vi "create_pattern.vi"(7 "sampling rate":dbl[unit], 8 "error in (no error)":errorcluster, 9 "duration":dbl[unit], 10 "amplitude":dbl, 11 "frequency":dbl[unit]=20000.0) -> (0 "error out":errorcluster, 2 "pattern values":dbl[](array[numeric]))   [LabVIEW 2010]
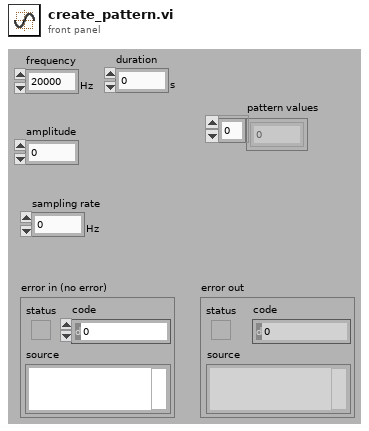
[diagram p1: front panel]
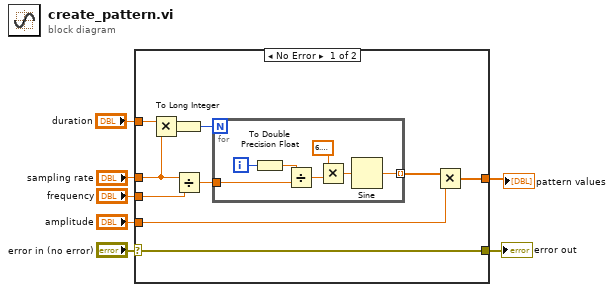
[diagram p0: block diagram]
diagram:
  n1 = case shown="No Error" "error in (no error)" {
    selector: "error in (no error)" -> [w17 w25]
    tunnel: [w17 w25] -> w6
    tunnel: "amplitude" -> [w16 _]
    tunnel: "frequency" -> [w13 _]
    tunnel: [w14 _] -> w3
    tunnel: "sampling rate" -> [w10 _]
    tunnel: "duration" -> [w11 _]
    frame No Error {
      n2 = Multiply(x=w11, y=w10) -> (x*y=w9:dbl)
      n3 = To Long Integer(number=w9) -> (32bit integer=w8:i32)
      n4 = Divide(x=w10, y=w13) -> (x/y=w12:dbl)
      n5 = for {
        N: w8 -> [_]
        tunnel: [w19] -> w15 mode=indexing
        tunnel: w12 -> [w18]
        i -> [w24]
        n6 = To Double Precision Float(number=w24) -> (double precision float=w23:dbl)
        n7 = Divide(x=w23, y=w18) -> (x/y=w22:dbl)
        n8 = Multiply(x=6.283185307179586, y=w22) -> (x*y=w20:dbl)
        n9 = Sine(x=w20) -> (sin(x)=w19:dbl)
      }
      n10 = Multiply(x=w15, y=w16) -> (x*y=w14:dbl[])
    }
    frame Error {
    }
  }
  "error out" <- w6
  "pattern values" <- w3
